vi "Parallel cascade example.vi"() -> ()   [LabVIEW 2019]
uses:
  <vilib>/addons/Control Design/_Model Construction/Model Creation.llb/Model Creation SubVI/cd_Create Transfer Function Model.vi
  <vilib>/addons/Control Design/_Utility/Model Viewer.llb/Model Viewer SubVI/cd_Draw Transfer Function Equation (TF).vi
  <vilib>/addons/Control Design/_Model Interconnection/Model Interconnection.llb/Model Interconnection SubVI/cd_Parallel (TF and TF).vi
  <vilib>/addons/Control Design/_Model Construction/NI_LinSys_Model Creation.lvlib
  <vilib>/addons/Control Design/_Utility/NI_CD_Model Viewer.lvlib
  <vilib>/addons/Control Design/_Model Interconnection/NI_CD_Model Interconnection.lvlib
panel:
  out "G2(s)":picture
  out "G1(s)":picture
  in  "Denominator 2":dbl[](array[numeric]) format="%#.5g"
  in  "Numerator 2":dbl[](array[numeric]) format="%#.5g"
  out "G1(s)+G2(s)":picture
  in  "Denominator":dbl[](array[numeric]) format="%#.5g"
  in  "Numerator":dbl[](array[numeric]) format="%#.5g"
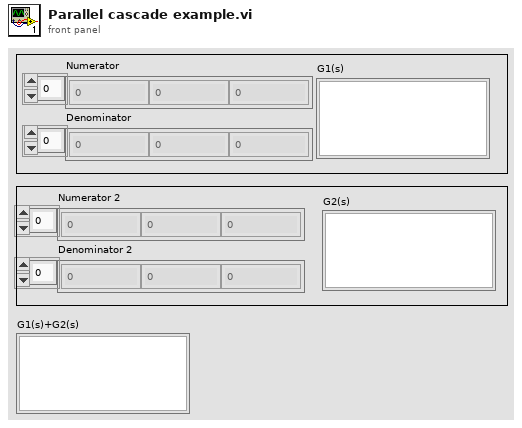
[diagram p1: front panel]
types:
  T1 = typedef "NI_LinSys_Model Typedefs.lvlib/CD Transfer Function Model (MIMO).ctl" = cluster{"properties":T2, "transfer function(s)":T3[][]}
  T2 = typedef "NI_LinSys_Model Typedefs.lvlib/CD General Elements.ctl" = cluster{"Model name":string, "Input names":string[], "Output names":string[], "Input Delays":dbl[], "Output Delays":dbl[], "Sampling Time":dbl, "Notes":string}
  T3 = typedef "NI_LinSys_Model Typedefs.lvlib/CD Transfer Function Model (SISO).ctl" = cluster{"Numerator":dbl[], "Denominator":dbl[], "delay":dbl}
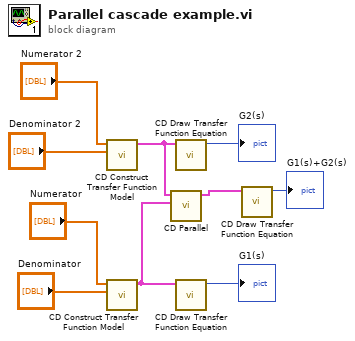
[diagram p0: block diagram]
diagram:
  n1 = call-poly <vilib>:"CD Construct Transfer Function Model.vi"("Denominator"="Denominator 2", "Numerator"="Numerator 2") -> ("Transfer Function Model"=w2:T1)  [unwired: 8 in, 1 out]
  n2 = call-poly <vilib>:"CD Construct Transfer Function Model.vi"("Denominator"="Denominator", "Numerator"="Numerator") -> ("Transfer Function Model"=w1:T1)  [unwired: 8 in, 1 out]
  n3 = call-poly <vilib>:"CD Parallel.vi"("Model 2"=w1, "Model 1"=w2) -> ("Parallel Model"=w3:T1)  [unwired: 8 in, 1 out]
  n4 = call-poly <vilib>:"CD Draw Transfer Function Equation.vi"("Transfer Function Model"=w2) -> ("Equation"=→"G2(s)":picture)  [unwired: 8 in, 2 out]
  n5 = call-poly <vilib>:"CD Draw Transfer Function Equation.vi"("Transfer Function Model"=w1) -> ("Equation"=→"G1(s)":picture)  [unwired: 8 in, 2 out]
  n6 = call-poly <vilib>:"CD Draw Transfer Function Equation.vi"("Transfer Function Model"=w3) -> ("Equation"=→"G1(s)+G2(s)":picture)  [unwired: 8 in, 2 out]
